vi "Fault Matrix 2 Bit.vi"(10 "Within Limits":T1) -> (2 "No Faults":bool)   [LabVIEW 2013]
uses:
  Within Limits Matrix.ctl
  Actuator Faults.ctl
  Cart Disp Faults.ctl
  Cart Force Faults.ctl
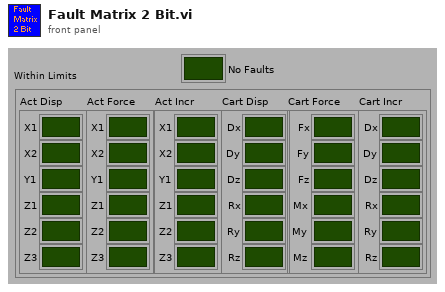
[diagram p1: front panel]
types:
  T1 = typedef "Within Limits Matrix.ctl" = cluster{"Act Disp":T2, "Act Force":T2, "Act Incr":T2, "Cart Disp":T3, "Cart Force":T4, "Cart Incr":T3}
  T2 = typedef "Actuator Faults.ctl" = cluster{"X1":bool, "X2":bool, "Y1":bool, "Z1":bool, "Z2":bool, "Z3":bool}
  T3 = typedef "Cart Disp Faults.ctl" = cluster{"Dx":bool, "Dy":bool, "Dz":bool, "Rx":bool, "Ry":bool, "Rz":bool}
  T4 = typedef "Cart Force Faults.ctl" = cluster{"Fx":bool, "Fy":bool, "Fz":bool, "Mx":bool, "My":bool, "Mz":bool}
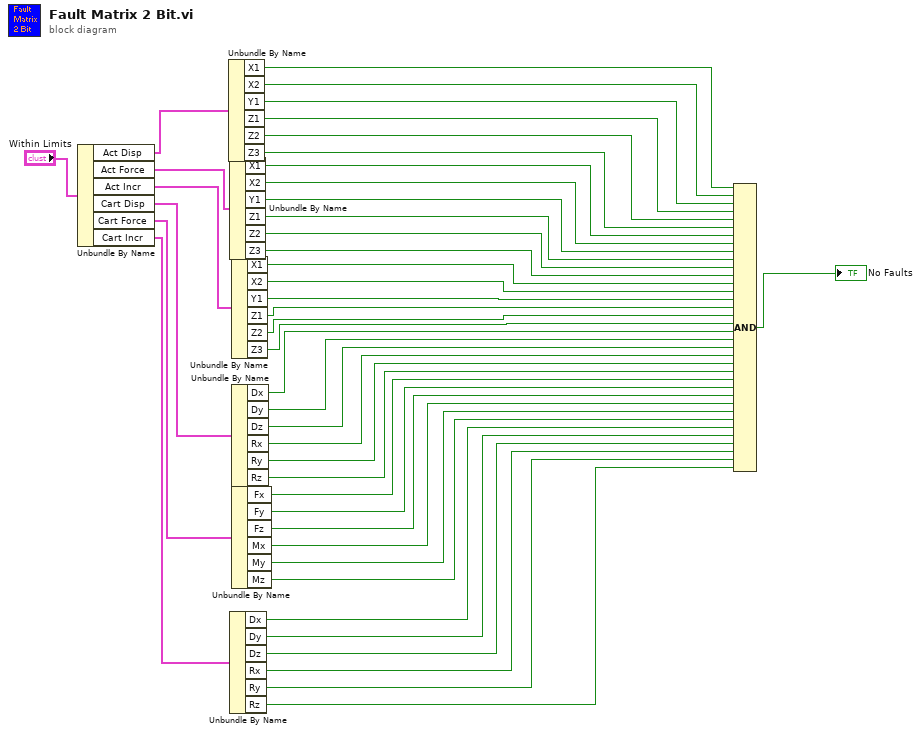
[diagram p0: block diagram]
diagram:
  n1 = Unbundle By Name("Within Limits") -> ("Act Disp"=w43:T2, "Act Force"=w42:T2, "Act Incr"=w7:T2, "Cart Disp"=w41:T3, "Cart Force"=w40:T4, "Cart Incr"=w14:T3)
  n2 = Unbundle By Name(w43) -> ("X1"=w39:bool, "X2"=w38:bool, "Y1"=w37:bool, "Z1"=w36:bool, "Z2"=w35:bool, "Z3"=w34:bool)
  n3 = Unbundle By Name(w42) -> ("X1"=w33:bool, "X2"=w32:bool, "Y1"=w31:bool, "Z1"=w30:bool, "Z2"=w29:bool, "Z3"=w28:bool)
  n4 = Unbundle By Name(w14) -> ("Dx"=w13:bool, "Dy"=w12:bool, "Dz"=w11:bool, "Rx"=w10:bool, "Ry"=w9:bool, "Rz"=w8:bool)
  n5 = Unbundle By Name(w7) -> ("X1"=w6:bool, "X2"=w5:bool, "Y1"=w4:bool, "Z1"=w3:bool, "Z2"=w2:bool, "Z3"=w1:bool)
  n6 = Unbundle By Name(w41) -> ("Dx"=w27:bool, "Dy"=w26:bool, "Dz"=w25:bool, "Rx"=w24:bool, "Ry"=w23:bool, "Rz"=w22:bool)
  n7 = Unbundle By Name(w40) -> ("Fx"=w21:bool, "Fy"=w20:bool, "Fz"=w19:bool, "Mx"=w18:bool, "My"=w17:bool, "Mz"=w16:bool)
  n8 = Compound Arithmetic op=AND(w39, w38, w37, w36, w35, w34, w33, w32, w31, w30, w29, w28, w6, w5, w4, w3, w2, w1, w27, w26, w25, w24, w23, w22, w21, w20, w19, w18, w17, w16, w13, w12, w11, w10, w9, w8) -> (→"No Faults":bool)
